vi "N Channel 1 Sample - Auto Indexing.vi"() -> ()   [LabVIEW 2026, in "synnax_clib.lvlib"]
uses:
  lvlib/synnax_clib.lvlib
  lvlib/typedefs/connection_config.ctl
  lvlib/classes/Client/Private/synnax channel retrieve keys Array.vi
  lvlib/classes/Writer/Private/synnax writer open Array.vi
  lvlib/classes/Writer/Private/Writes/I32/Write NCh 1Samp (I32).vi
  lvlib/classes/Synnax Writer.lvclass
  lvlib/classes/Client/Synnax Client.lvclass
panel:
  in  "Channels":string[](array[numeric])=["my_i32_ch1", "my_i32_ch2", "my_i32_ch3", "my_i32_ch4"]
  in  "Stop":bool
  out "error out":errorcluster
  in  "Connection Config":T1={"host"="localhost", "port"=9090, "username"="synnax", "password"="seldon"}
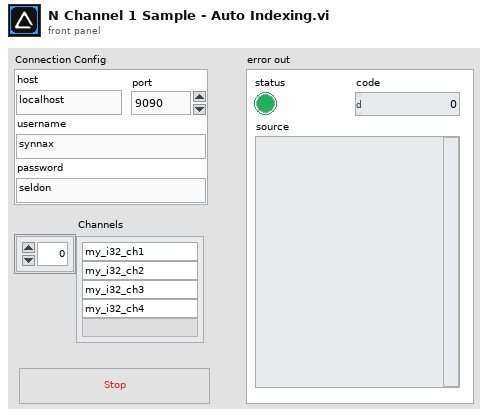
[diagram p1: front panel]
types:
  T1 = typedef "synnax_clib.lvlib/connection_config.ctl" = cluster{"host":string, "port":u16, "username":string, "password":string}
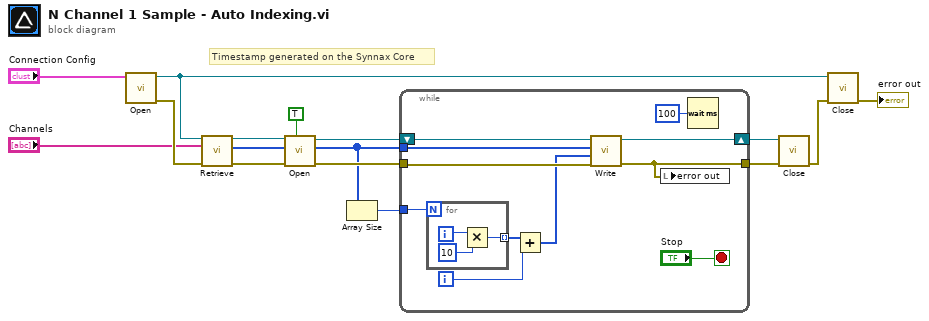
[diagram p0: block diagram]
diagram:
  # "Timestamp generated on the Synnax Core"
  n1 = call "Open.vi"("Connection Config"="Connection Config") -> ("error out"=w11:errorcluster, "Synnax Client out"=w13:refnum<class "Synnax Client.lvclass">)  [unwired: 9 in]
  n2 = call-poly "Retrieve.vi"("Synnax Client in"=w13, "channel names"="Channels", "error in"=w11) -> ("Synnax Client out"=w7:refnum<class "Synnax Client.lvclass">, "channel keys"=w5:u32[], "error out"=w15:errorcluster)  [unwired: 8 in, 2 out]
  n3 = call-poly "Open.vi"("auto_index (F)"=TRUE, "error in"=w15, "channels in"=w5, "Synnax Client in"=w7) -> ("error out"=w8:errorcluster, "channels out"=w3:u32[], "writer out"=w10:refnum<class "Synnax Writer.lvclass">)  [unwired: 5 in]
  n4 = Array Size(array=w3) -> (size(s)=w2:i32)
  n5 = while {
    shift-right: [w26] -> w9
    shift-left: w10 -> [w27]
    tunnel: w8 -> [w25]
    tunnel: [w22] -> w16
    tunnel: w3 -> [w20]
    tunnel: w2 -> [w19]
    i -> [w17]
    stop <- "Stop" stop-if-true
    n6 = for {
      N: w19 -> [_]
      tunnel: [w29] -> w23 mode=indexing
      i -> [w30]
      n7 = Multiply(x=w30, y=10) -> (x*y=w29:i32)
    }
    n8 = Add(x=w23, y=w17) -> (x+y=w18:i32[])
    n9 = call-poly "Write.vi"("error in"=w25, "data"=w18, "channels"=w20, "Writer"=w27) -> ("error out"=w22:errorcluster, "Writer Out"=w26:refnum<class "Synnax Writer.lvclass">)  [unwired: 6 in]
    n10 = local write "error out"(w22) -> ()
    n11 = Wait (ms)(milliseconds to wait=u32 100) -> ()  [unwired: 1 out]
  }
  n12 = call "Close.vi"("error in"=w16, "writer"=w9) -> ("error out"=w12:errorcluster)  [unwired: 9 in]
  n13 = call "Close.vi"("error in"=w12, "Synnax Client in"=w13) -> ("error out"=→"error out":errorcluster)  [unwired: 9 in]
